vi "--direct.vi"(7 "Actor in":refnum<class "Actor.lvclass">, 10 "Pump State":bool) -> (0 "Error out":errorcluster, 5 "Actor out":refnum<class "Actor.lvclass">)   [LabVIEW 2025, in "Update Pump State Msg.lvlib"]
uses:
  Update Pump State Msg.lvlib
  <vilib>/Nathan Davis/jettl/jettl/jettl/Actor/Actor/Actor.lvclass
  Update Pump State Msg/Update Pump State Msg.lvclass
  <vilib>/Nathan Davis/jettl/jettl/jettl/Actor/Actor.lvlib
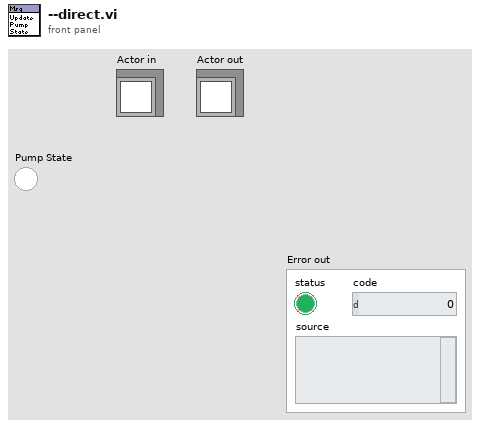
[diagram p1: front panel]
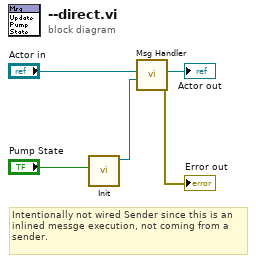
[diagram p0: block diagram]
diagram:
  # "Intentionally not wired Sender since this is an inlined messge execution, not coming from a sender."
  n1 = call "Init.vi"("Pump State"="Pump State") -> ("Update Pump State Msg out"=w1:refnum<class "Update Pump State Msg.lvclass">)  [unwired: 10 in]
  n2 = call <vilib>:"Msg Handler.vi"("Msg"=w1, "Actor in"="Actor in") -> ("Error out"=→"Error out":errorcluster, "Actor out"=→"Actor out":refnum<class "Actor.lvclass">)  [unwired: 8 in]
